vi "Read_Daxsonics_3Pulsers.vi"(10 "Num Channels":i32=5) -> (0 "Dax Values":T1 {"Freq (MHz)" items=["50"=50, "45"=45, "40"=40, "35"=35, "30"=30, "25"=25, "20"=20, "18"=18, "17"=17, "16"=16, "15"=15, "14"=14, "12"=12, "10"=10, "8"=8, "6"=6, "5"=5, "4"=4]; "Voltage (V)" items=["190"=190, "180"=180, "170"=170, "160"=160, "150"=150, "140"=140, "130"=130, "120"=120, "110"=110, "100"=100, "95"=95, "90"=90, "85"=85, "80"=80, "75"=75, "70"=70, "65"=65, "60"=60, "55"=55, "50"=50, "45"=45, "40"=40, "35"=35, "30"=30, "25"=25, "20"=20, "15"=15, "10"=10, "5"=5, "0"=0]; "Gain (dB)" items=["67"=67, "64"=64, "61"=61, "58"=58, "55"=55, "52"=52, "49"=49, "46"=46, "43"=43, "40"=40, "37"=37, "34"=34, "31"=31, "28"=28, "25"=25, "22"=22]}, 1 "Freq (MHz)":u16=5, 2 "Voltage (V)":u16, 3 "Gains":u16[](array[numeric]), 5 "Trigger Ext(T)/Int(F)":bool, 6 "HI(T)/LO(F) +12 dB":bool=TRUE, 7 "Trigger Rising (T)/Falling (F)":bool=TRUE)   [LabVIEW 2022 SP3]
uses:
  Dax_Control_Cluster.ctl
  PulserGlobals.vi
panel:
  out "Array 2":string[](array[string])
  out "Array":errorcluster[](array[cluster])
  out "PRI":i32
  out "NUMTX":i32
  out "enable Table":i32[][](array[numeric])
  out "delay table":i32[][](array[numeric])
  # "time from Dax converted to frequencey for new dax"
  # "New Daxsonics"
  # "FREQ for new daxsonics is in fact a time value"
  # "Column is element #\n\nList of which xmit element active"
  # "Column is element #"
  # "Row is tx event\nOnly numtx are transmitted"
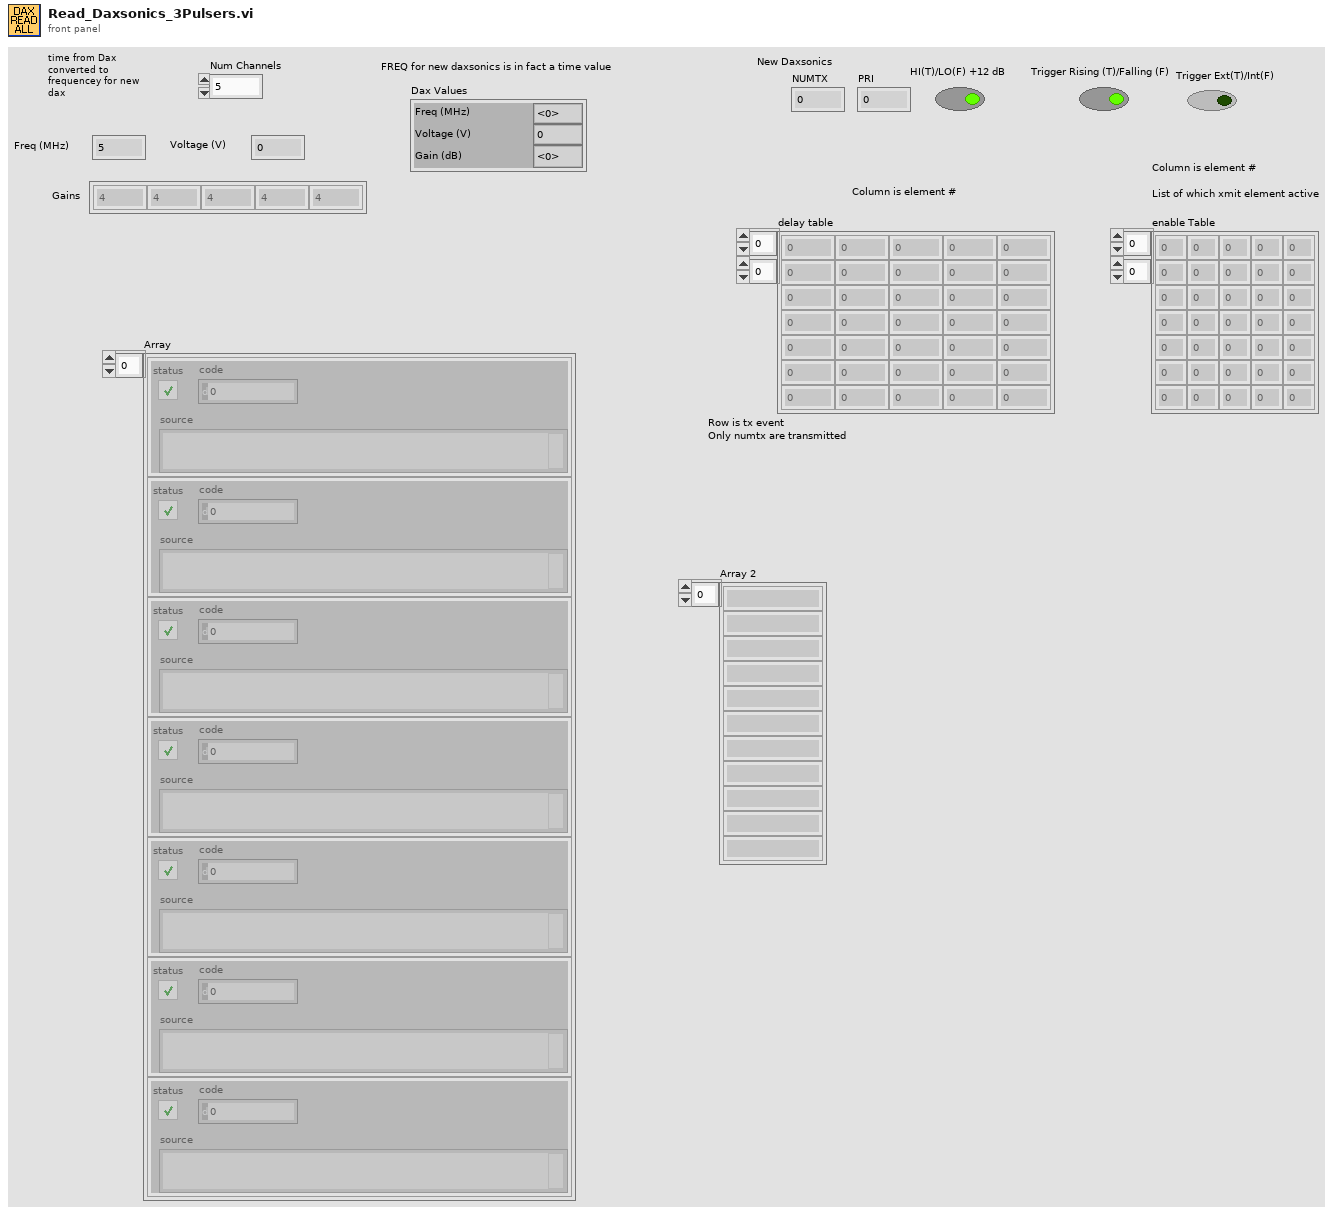
[diagram p1: front panel]
types:
  T1 = typedef "Dax_Control_Cluster.ctl" = cluster{"Freq (MHz) ":u16, "Voltage (V)":u16, "Gain (dB)":u16}
  T2 = typedef "Daxsonics_Pulsers.ctl" = enum16{"BP1", "BP2_A", "BP2_B", "10ERS8", "New2021"}
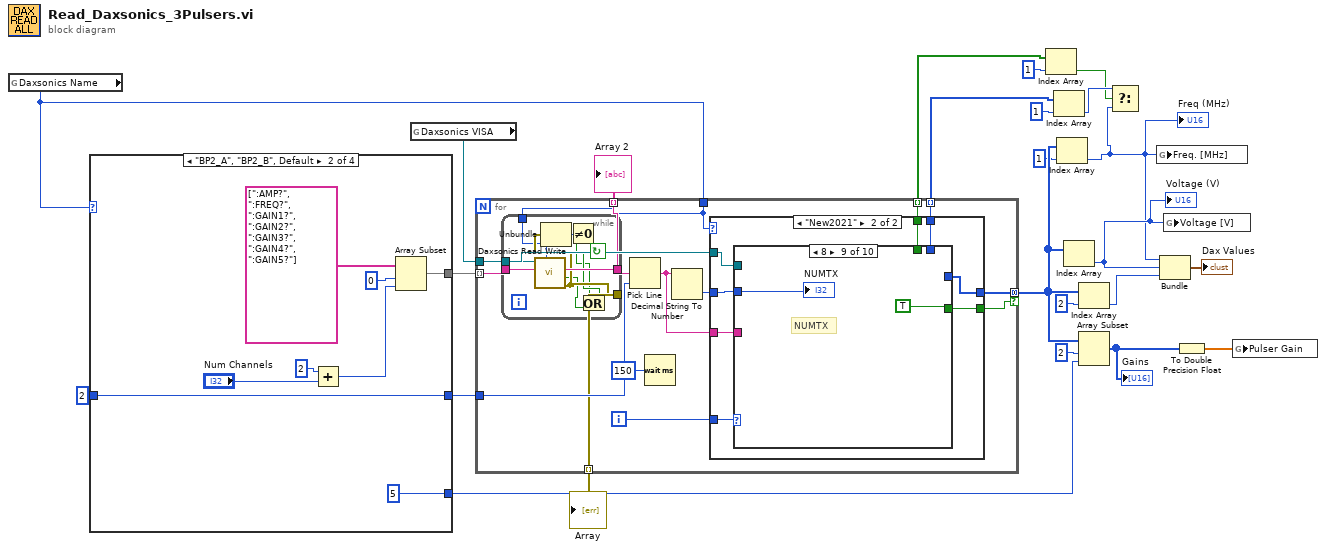
[diagram p0: block diagram]
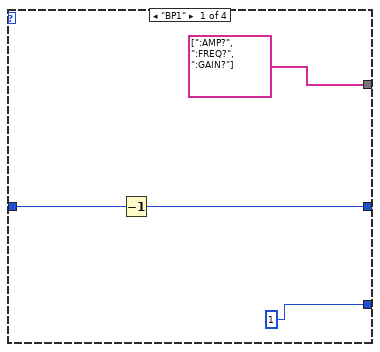
[diagram p2: hidden frame]
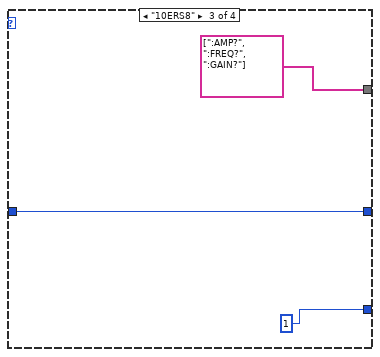
[diagram p3: hidden frame]
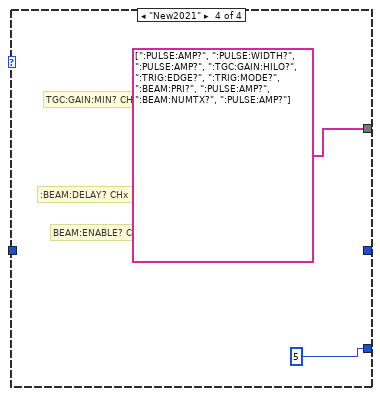
[diagram p4: hidden frame]
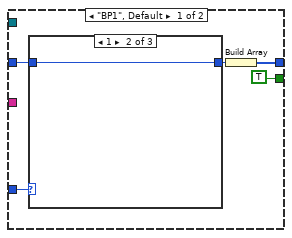
[diagram p5: hidden frame]
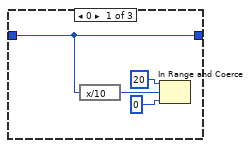
[diagram p6: hidden frame]
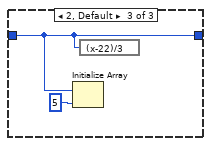
[diagram p7: hidden frame]
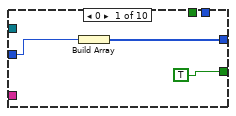
[diagram p8: hidden frame]
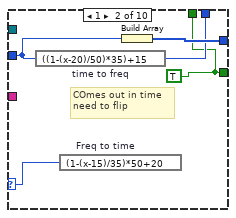
[diagram p9: hidden frame]
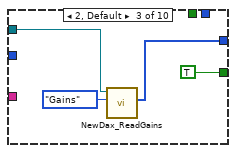
[diagram p10: hidden frame]
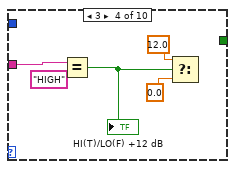
[diagram p11: hidden frame]
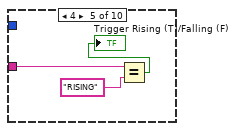
[diagram p12: hidden frame]
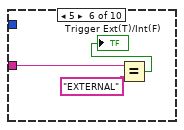
[diagram p13: hidden frame]
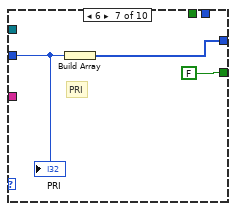
[diagram p14: hidden frame]
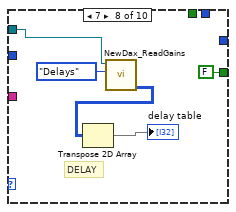
[diagram p15: hidden frame]
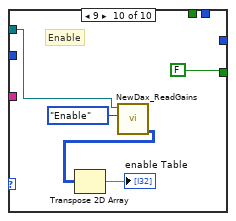
[diagram p16: hidden frame]
diagram:
  n1 = global read "PulserGlobals.vi" "Daxsonics Name"() -> (w12:T2)
  n2 = case shown="\"BP2_A\", \"BP2_B\", Default" w12 {
    tunnel: [string[] [":AMP?", ":FREQ?", ":GAIN?"] w35 string[] [":AMP?", ":FREQ?", ":GAIN?"] string[] [":PULSE:AMP?", ":PULSE:WIDTH?", ":PULSE:AMP?", ":TGC:GAIN:HILO?", ":TRIG:EDGE?", ":TRIG:MODE?", ":BEAM:PRI?", ":PULSE:AMP?", ":BEAM:NUMTX?", ":PULSE:AMP?"]] -> w23
    tunnel: [w26 w30 w38 _] -> w15
    tunnel: 2 ("line index") -> [w27 w30 w38 _]
    tunnel: [1 ("length") 5 ("length") 1 ("length") 5 ("length")] -> w10
    frame "BP1" {
      n3 = Decrement(x=w27) -> (x-1=w26:i32)
    }
    frame "BP2_A", "BP2_B", Default {
      n4 = Add(x=2, y="Num Channels") -> (x+y=w32:i32)
      n5 = Array Subset(array=string[] [":AMP?", ":FREQ?", ":GAIN1?", ":GAIN2?", ":GAIN3?", ":GAIN4?", ":GAIN5?"], index=0, length=w32) -> (w35:string[])
    }
    frame "10ERS8" {
    }
    frame "New2021" {
      # "BEAM:ENABLE? CHx"
      # ":BEAM:DELAY? CHx"
      # "TGC:GAIN:MIN? CHx"
    }
  }
  n6 = global read "PulserGlobals.vi" "Daxsonics VISA"() -> (w13:refnum<visa-resource-name>)
  n7 = for {
    tunnel: w23 -> [w53] mode=indexing
    tunnel: w13 -> [w49]
    tunnel: [w52] -> w22 mode=concatenating if=w50
    tunnel: w15 -> [w51]
    tunnel: w12 -> [w42]
    tunnel: [w48] -> w8 mode=indexing
    tunnel: [w47] -> w5 mode=indexing
    tunnel: [w45] -> w2 mode=indexing
    tunnel: [w44] -> w1 mode=indexing
    i -> [w55]
    n8 = while {
      tunnel: w49 -> [w63]
      tunnel: [w61] -> w45
      tunnel: w53 -> [w64]
      tunnel: [w62] -> w44
      tunnel: w42 -> [w56]
      stop <- w58 continue-if-true
      n9 = call "Daxsonics Read Write.vi"("Daxsonics Name"=w56, "write buffer"=w64, "VISA resource name"=w63) -> ("error out"=w61:errorcluster, "Success?"=w59:bool, "read buffer"=w62:string)  [unwired: 6 in]
      n10 = Unbundle(w61) -> ("code"=w60:i32)  [unwired: 2 out]
      n11 = Not Equal To 0?(x=w60) -> (x != 0?=w57:bool)
      n12 = Or(x=w57, y=w59) -> (x .or. y?=w58:bool)
    }
    n13 = Pick Line(multi-line string=w44, line index=w51) -> (output string=w46:string)  [unwired: 1 in]
    n14 = Wait (ms)(milliseconds to wait=u32 150) -> ()  [unwired: 1 out]
    n15 = Decimal String To Number(string=w46) -> (number=w54:i32)  [unwired: 2 in, 1 out]
    n16 = case shown="\"New2021\"" w42 {
      tunnel: w55 -> [w69 w80]
      tunnel: w54 -> [w68 w84]
      tunnel: [w65 w83] -> w52
      tunnel: [TRUE w82] -> w50
      tunnel: w46 -> [_ w81]
      tunnel: w49 -> [_ w79]
      tunnel: [_ w78] -> w48
      tunnel: [_ w77] -> w47
      frame "BP1", Default {
        n17 = case shown="1" w69 {
          tunnel: w68 -> [w70 w74 w75]
          tunnel: [w70 w74 w75] -> w67
          frame 0 {
            n18 = expression code="x/10"(w70) -> (w73:i32)
            n19 = In Range and Coerce(upper limit=20, x=w73, lower limit=0) -> ()  [unwired: 2 out]
          }
          frame 1 {
          }
          frame 2, Default {
            n20 = Initialize Array(w75, 5 ("dimension size")) -> ()  [unwired: 1 out]
            n21 = expression code="(x-22)/3"(w75) -> ()  [unwired: 1 out]
          }
        }
        n22 = Build Array(w67) -> (w65:i32[])
      }
      frame "New2021" {
        n23 = case shown="8" w80 {
          selector: w80 -> [_ w91 _ _ _ _ _ _ _ _]
          tunnel: w84 -> [w86 w90 _ _ _ _ w110 _ w117 _]
          tunnel: [w85 w92 w94 _ _ _ w108 _ _ _] -> w83
          tunnel: [TRUE w88 TRUE _ _ _ FALSE FALSE TRUE FALSE] -> w82
          tunnel: w81 -> [_ _ _ w100 w104 w107 _ _ _ _]
          tunnel: w79 -> [_ _ w93 _ _ _ _ w113 _ w120]
          tunnel: [_ w89 _ _ _ _ _ _ _ _] -> w78
          tunnel: [_ w88 _ _ _ _ _ _ _ _] -> w77
          frame 0 {
            n24 = Build Array(w86) -> (w85:i32[])
          }
          frame 1 {
            w88 = TRUE
            # "COmes out in time\nneed to flip"
            n25 = expression code="((1-(x-20)/50)*35)+15" "time to freq"(w90) -> (w89:i32)
            n26 = expression code="(1-(x-15)/35)*50+20" "Freq to time"(w91) -> ()  [unwired: 1 out]
            n27 = Build Array(w90) -> (w92:i32[])
          }
          frame 2, Default {
            n28 = call "NewDax_ReadGains.vi"("Ch Option"=enum16{"Gains", "Delays", "Slope", "Enable"}."Gains", "Daxsonics VISA"=w93) -> ("Values Out"=w94:i32[])  [unwired: 8 in, 1 out]
          }
          frame 3 {
            n29 = Equal?(x=w100, y="HIGH") -> (x = y?=w97:bool)
            "HI(T)/LO(F) +12 dB" <- w97
            n30 = Select(t=12.0, s=w97, f=0.0 ("t")) -> ()  [unwired: 1 out]
          }
          frame 4 {
            n31 = Equal?(x=w104, y="RISING") -> (x = y?=→"Trigger Rising (T)/Falling (F)":bool)
          }
          frame 5 {
            n32 = Equal?(x=w107, y="EXTERNAL") -> (x = y?=→"Trigger Ext(T)/Int(F)":bool)
          }
          frame 6 {
            # "PRI"
            n33 = Build Array(w110) -> (w108:i32[])
            "PRI" <- w110
          }
          frame 7 {
            # "DELAY"
            n34 = call "NewDax_ReadGains.vi"("Ch Option"=enum16{"Gains", "Delays", "Slope", "Enable"}."Delays", "Daxsonics VISA"=w113) -> ("Array"=w112:i32[][])  [unwired: 8 in, 1 out]
            n35 = Transpose 2D Array(2D array=w112) -> (transposed array=→"delay table":i32[][])
          }
          frame 8 {
            # "NUMTX"
            "NUMTX" <- w117
          }
          frame 9 {
            # "Enable"
            n36 = call "NewDax_ReadGains.vi"("Ch Option"=enum16{"Gains", "Delays", "Slope", "Enable"}."Enable", "Daxsonics VISA"=w120) -> ("Array"=w119:i32[][])  [unwired: 8 in, 1 out]
            n37 = Transpose 2D Array(2D array=w119) -> (transposed array=→"enable Table":i32[][])
          }
        }
      }
    }
  }
  "Array" <- w2
  "Array 2" <- w1
  n38 = Index Array(array=w5, index=1) -> (element=w4:bool)
  n39 = Index Array(array=w8, index=1) -> (element=w7:i32)
  n40 = Index Array(array=w22, index=1) -> (element=w3:i32)
  "Freq (MHz)" <- w3
  n41 = Index Array(array=w22) -> (element=w11:i32)  [unwired: 1 in]
  "Voltage (V)" <- w11
  n42 = Index Array(array=w22, index=2) -> (element=w21:i32)
  n43 = Array Subset(array=w22, index=2, length=w10) -> (w17:i32[])
  "Gains" <- w17
  n44 = Select(t=w7, s=w4, f=w3) -> ()  [unwired: 1 out]
  n45 = global write "PulserGlobals.vi" "Freq. [MHz]"(w3) -> ()
  n46 = Bundle(w3, w11, w21) -> (→"Dax Values":cluster{i32, i32, i32})  [unwired: 1 in]
  n47 = global write "PulserGlobals.vi" "Voltage [V]"(w11) -> ()
  n48 = To Double Precision Float(number=w17) -> (double precision float=w16:dbl[])
  n49 = global write "PulserGlobals.vi" "Pulser Gain"(w16) -> ()
